vi "myRIO_BRig_RT_dataCurrent_laser1_triggered_Sel.vi"() -> (2 "output_laser1_triggered_Selection":i32)   [LabVIEW 2014]
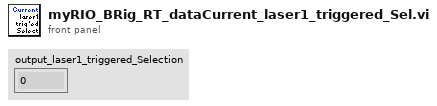
[diagram p1: front panel]
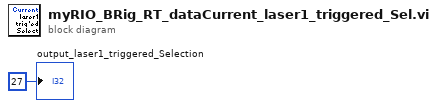
[diagram p0: block diagram]
diagram:
  "output_laser1_triggered_Selection" <- 27 ("output_iBlock")
